vi "Status_write_VS.vi"(8 "error_in":errorcluster, 9 "Status_Cluster_in":T1, 10 "Ref":T4) -> (0 "error_out":errorcluster, 1 "Status_Cluster_out":T1)   [LabVIEW 2020, in "Vires VTD Engine.lvlib"]
doc: "Updates the Status changes and writes them to VeriStand"
uses:
  Vires VTD Engine.lvlib
  Type/Status_Cluster.ctl
  Type/ConnectionStatus.ctl
  Type/CaseSelection.ctl
  <vilib>/NI/NIVS Inline Async API/_Data Access Engine/Data Access Engine/Types/ReadWrite.DVR.ctl
  <vilib>/NI/NIVS Inline Async API/_Data Access Engine/Access Type Classes/ReadWrite/ReadWrite.lvclass
  <vilib>/NI/NIVS Inline Async API/_Data Access Engine/Access Type Classes/ReadWrite/ReadWrite.lvclass/ReadWrite.ctl
  <vilib>/NI/NIVS Inline Async API/_Data Access Engine/Data Access Engine/Methods/ReadWrite.Data.Write.vi
  <vilib>/NI/NIVS Inline Async API/_Data Access Engine/Access Type Classes/ReadWrite/ReadWrite.ProcessData.Write.vi
  <vilib>/NI/NIVS Inline Async API/_Data Access Engine/Access Type Classes/ReadWrite/ReadWrite.ProcessData.Buffer.vi
  <vilib>/NI/NIVS Inline Async API/_Data Access Engine/Access Type Classes/ReadWrite/ReadWrite.ProcessData.Commit.vi
  <vilib>/NI/NIVS Inline Async API/_Data Access Engine/Data Access Engine/Data Access Engine.lvclass
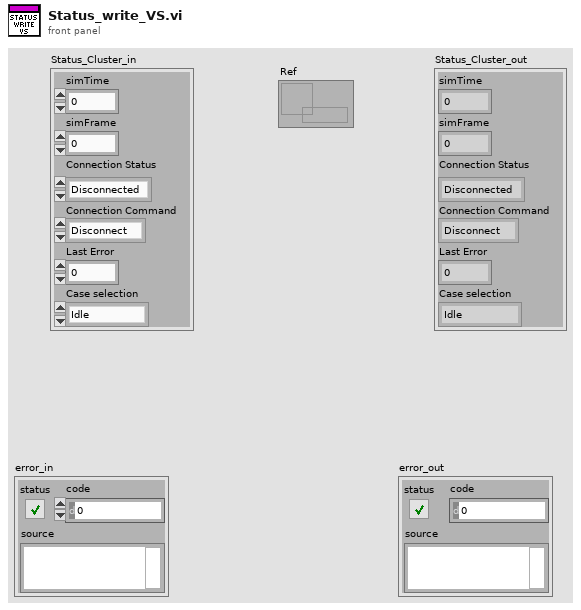
[diagram p1: front panel]
types:
  T1 = typedef "Vires VTD Engine.lvlib/Status_Cluster.ctl" = cluster{"simTime":dbl, "simFrame":dbl, "Connection Status":T2, "Connection Command":enum16{"Disconnect", "Connect"}, "Last Error":i32, "Case selection":T3}
  T2 = typedef "Vires VTD Engine.lvlib/ConnectionStatus.ctl" = enum16{"Disconnected", "Connected"}
  T3 = typedef "Vires VTD Engine.lvlib/CaseSelection.ctl" = enum32{"Idle", "Connecting", "Disconnecting", "Read/Write"}
  T4 = typedef "Data Access Engine.lvlib/Data Access Engine.lvclass/ReadWrite.DVR.ctl" = refnum<data-value>
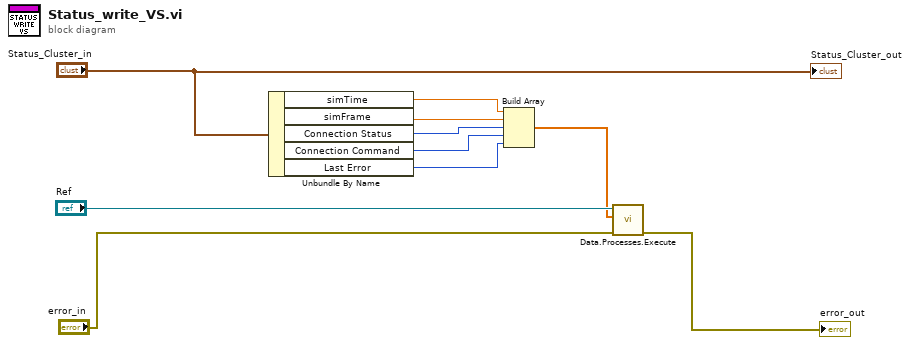
[diagram p0: block diagram]
diagram:
  n1 = Unbundle By Name("Status_Cluster_in") -> ("simTime"=w6:dbl, "simFrame"=w5:dbl, "Connection Status"=w4:T2, "Connection Command"=w3:enum16{"Disconnect", "Connect"}, "Last Error"=w2:i32)
  n2 = Build Array(w6, w5, w4, w3, w2) -> (w7:dbl[])
  n3 = call-poly <vilib>:"Data.Processes.Execute.vi"("error in (no error)"="error_in", "Values"=w7, "Ref"="Ref") -> ("error out"=→"error_out":errorcluster)  [unwired: 8 in]
  "Status_Cluster_out" <- "Status_Cluster_in"
